vi "Bisect Angle.vi"   [LabVIEW 2017, in "NI_AAL_Angle.lvlib"]
doc: "Calculates the angle that bisects the start angle and the end angle into two equal parts.\n\nWire data to any of the angle inputs to determine the polymorphic instance to use or manually select the instance."
uses:
  <vilib>/Analysis/NI_AAL_Angle.lvlib
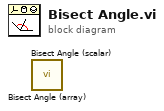
[diagram p0: block diagram]
diagram:
  n1 = call <vilib>:"Bisect Angle (array).vi"() -> ()  [unwired: 10 in, 2 out]
  n2 = call <vilib>:"Bisect Angle (scalar).vi"() -> ()  [unwired: 10 in, 2 out]
